vi "Voltage (Read).vi"(6 "ISOBUS address":T3=-1 caption="ISOBUS address (-1)", 8 "error in":errorcluster, 11 "Mercury Reference In":T4) -> (0 "error out":errorcluster, 1 "Unit":T1, 2 "Voltage":dbl, 3 "Mercury Reference Out":T4, 4 "Valid?":T2)   [LabVIEW 2018, in "Mercury iXX.lvlib" / "Temperature.lvlib"]
doc: "Acquire the most recent voltage reading."
uses:
  Temperature.lvlib
  Controls/Mercury Reference.ctl
  Controls/Comms Transport Layer.ctl
  Private/Controls/Query Dynamic Reference.ctl
  Controls/ISOBus Address.ctl
  Controls/Is Valid LED.ctl
  Controls/Unit String.ctl
  Private/Controls/Command Verbs.ctl
  Mercury iXX.lvlib
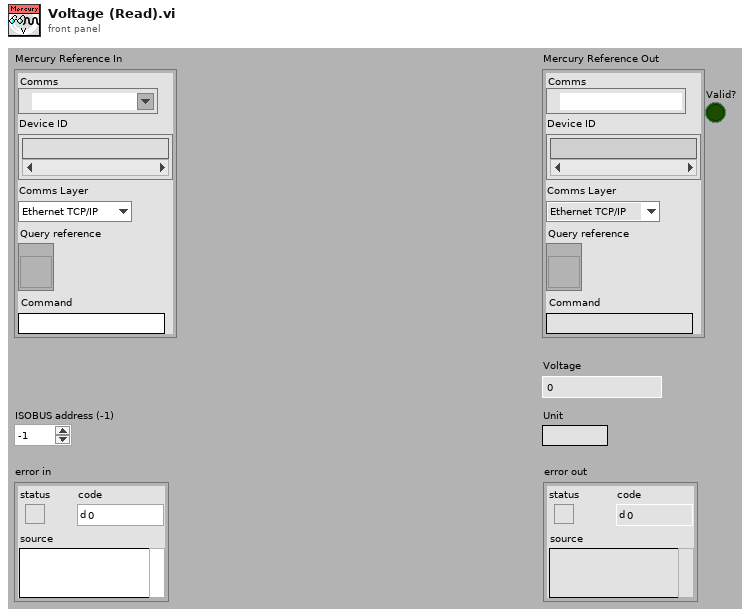
[diagram p1: front panel]
types:
  T1 = typedef "Mercury iXX.lvlib/Unit String.ctl" = string
  T2 = typedef "Mercury iXX.lvlib/Is Valid LED.ctl" = bool
  T3 = typedef "Mercury iXX.lvlib/ISOBus Address.ctl" = i32
  T4 = typedef "Mercury iXX.lvlib/Mercury Reference.ctl" = cluster{"Comms":refnum<visa-resource-name>, "Device ID":string[], "Comms Layer":T5, "Command":string, "Query reference":T6}
  T5 = typedef "Mercury iXX.lvlib/Comms Transport Layer.ctl" = enum16{"Ethernet TCP/IP", "USB", "ISOBus - RS-232", "GPIB"}
  T6 = typedef "Mercury iXX.lvlib/Query Dynamic Reference.ctl" = refnum<vi>
  T7 = typedef "Mercury iXX.lvlib/Command Verbs.ctl" = string
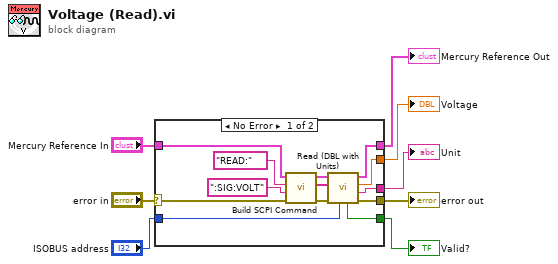
[diagram p0: block diagram]
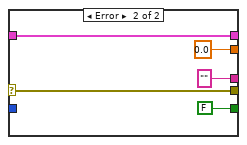
[diagram p2: hidden frame]
diagram:
  n1 = case shown="No Error" "error in" {
    selector: "error in" -> [w9 w26]
    tunnel: [w17 w25] -> w8
    tunnel: [w16 0.0 ("Data (Dbl)")] -> w7
    tunnel: [w15 T1 "" ("Unit")] -> w6
    tunnel: [w14 T2 FALSE ("Valid?")] -> w5
    tunnel: [w13 w26] -> w4
    tunnel: "Mercury Reference In" -> [w12 w25]
    tunnel: "ISOBUS address" -> [w11 _]
    frame No Error {
      n2 = call "Build SCPI Command.vi"("error in"=w9, "Noun(s)"=":SIG:VOLT" ("Command"), "Verb"=T7 "READ:", "Mercury Reference In"=w12) -> ("error out"=w21:errorcluster, "SCPI Message(s)"=w19:string[], "Mercury Reference Out"=w18:T4)  [unwired: 5 out]
      n3 = call "Read (DBL with Units).vi"("ISOBUS address"=w11, "error in"=w21, "SCPI Message(s)"=w19, "Mercury Reference In"=w18) -> ("error out"=w13:errorcluster, "Unit"=w15:T1, "Data (Dbl)"=w16:dbl, "Mercury Reference Out"=w17:T4, "Valid?"=w14:T2)  [unwired: 3 out]
    }
    frame Error {
    }
  }
  "Mercury Reference Out" <- w8
  "error out" <- w4
  "Voltage" <- w7
  "Valid?" <- w5
  "Unit" <- w6
